vi "Get AI Signal - All.vi"(0 "reference in":refnum<class "AI.lvclass">, 4 "Zero Threshold":dbl=0.001, 5 "error in (no error)":errorcluster) -> (11 "AI Signal is Zero":bool[](array[boolean]), 14 "reference out":refnum<class "AI.lvclass">, 16 "AI Readings":dbl[][](array[numeric]), 17 "AI Channel Averages":dbl[](array[numeric]), 18 "AI Chanel Standard Deviations":dbl[](array[numeric]), 19 "error out":errorcluster)   [LabVIEW 2017, in "AI.lvclass"]
uses:
  AI.lvclass
  <vilib>/Analysis/NI_AALBase.lvlib
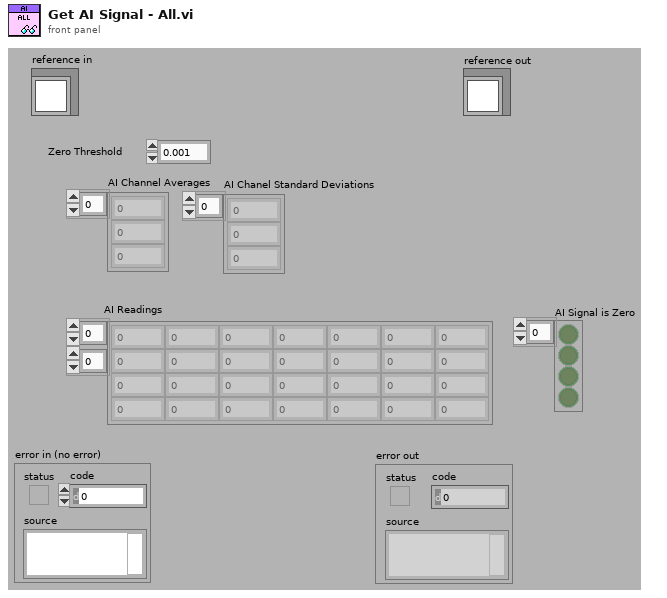
[diagram p1: front panel]
types:
  T1 = typedef "AI.lvclass/ObjectAttributes.ctl" = cluster{"AI Task":refnum<k21>, "AI On/Off Status":bool, "AI Sampling Rate (Samples/Seconds)":u32, "Number of AI Samples Per Channel":i32, "AI Voltage Range":u8, "AI Readings":dbl[][], "Number of AI Modules":i32, "Number of Total AI Channels":i32, "AI Module Names (NI-Max Name)":string[], "Number of Channels Per AI  Module":i32[], "AI VI Reference":refnum<vi>}
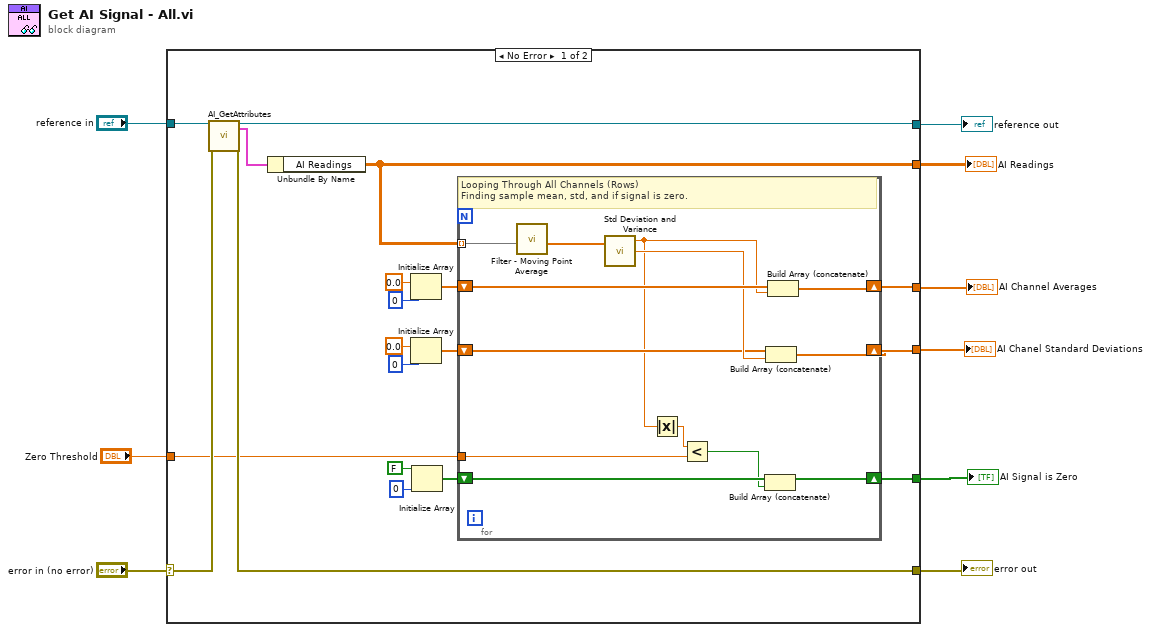
[diagram p0: block diagram]
diagram:
  n1 = case shown="No Error" "error in (no error)" {
    selector: "error in (no error)" -> [w27 w43]
    tunnel: [w25 w43] -> w8
    tunnel: [w26 w42] -> w6
    tunnel: "reference in" -> [w28 w42]
    tunnel: [w24 _] -> w5
    tunnel: [w23 _] -> w4
    tunnel: [w22 _] -> w3
    tunnel: [w21 _] -> w2
    tunnel: "Zero Threshold" -> [w10 _]
    frame No Error {
      n2 = call "AI_GetAttributes.vi"("reference in"=w28, "error in (no error)"=w27) -> ("reference out"=w26:refnum<class "AI.lvclass">, "Data"=w11:T1, "error out"=w25:errorcluster)  [unwired: 14 in, 1 out]
      n3 = Unbundle By Name(w11) -> ("AI Readings"=w24:dbl[][])
      n4 = Initialize Array(0.0 ("element"), 0 ("dimension size")) -> (w18:dbl[])
      n5 = Initialize Array(0.0 ("element"), 0 ("dimension size")) -> (w15:dbl[])
      n6 = Initialize Array(FALSE, 0 ("dimension size")) -> (w12:bool[])
      n7 = for {
        tunnel: w24 -> [w30] mode=indexing
        shift-right: [w40] -> w23
        shift-left: w18 -> [w41]
        shift-right: [w37] -> w22
        shift-left: w15 -> [w38]
        shift-right: [w34] -> w21
        shift-left: w12 -> [w36]
        tunnel: w10 -> [w31]
        # "Looping Through All Channels (Rows)\nFinding sample mean, std, and if signal is zero."
        n8 = call "Filter - Moving Point Average.vi"("Analog Signal"=w30) -> ("Filtered Analog Signal"=w29:dbl[])  [unwired: 10 in]
        n9 = call <vilib>:"Std Deviation and Variance.vi"("X"=w29) -> ("mean"=w33:dbl, "standard deviation"=w39:dbl)  [unwired: 1 in, 1 out]
        n10 = Absolute Value(x=w33) -> (abs(x)=w32:dbl)
        n11 = Less?(x=w32, y=w31) -> (x < y?=w35:bool)
        n12 = Build Array (concatenate)(w36, w35) -> (w34:bool[])
        n13 = Build Array (concatenate)(w38, w39) -> (w37:dbl[])
        n14 = Build Array (concatenate)(w41, w33) -> (w40:dbl[])
      }
    }
    frame Error {
    }
  }
  "error out" <- w8
  "reference out" <- w6
  "AI Readings" <- w5
  "AI Channel Averages" <- w4
  "AI Chanel Standard Deviations" <- w3
  "AI Signal is Zero" <- w2
